vi "情景列表删除.vi"(9 "删除节点":string, 10 "父节点（场景）":string, 11 "模式列表":T1(array[cluster])) -> (3 "模式列表-output":T1(array[cluster]))   [LabVIEW 2019]
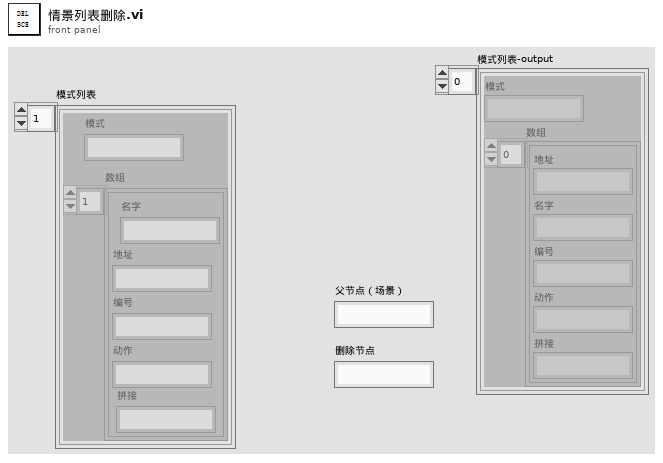
[diagram p1: front panel]
types:
  T1 = cluster{"模式":string, "数组":cluster{"地址":string, "名字":string, "编号":string, "动作":string, "拼接":string}[]}[]
  T2 = cluster{"模式":string, "数组":cluster{"地址":string, "名字":string, "编号":string, "动作":string, "拼接":string}[]}
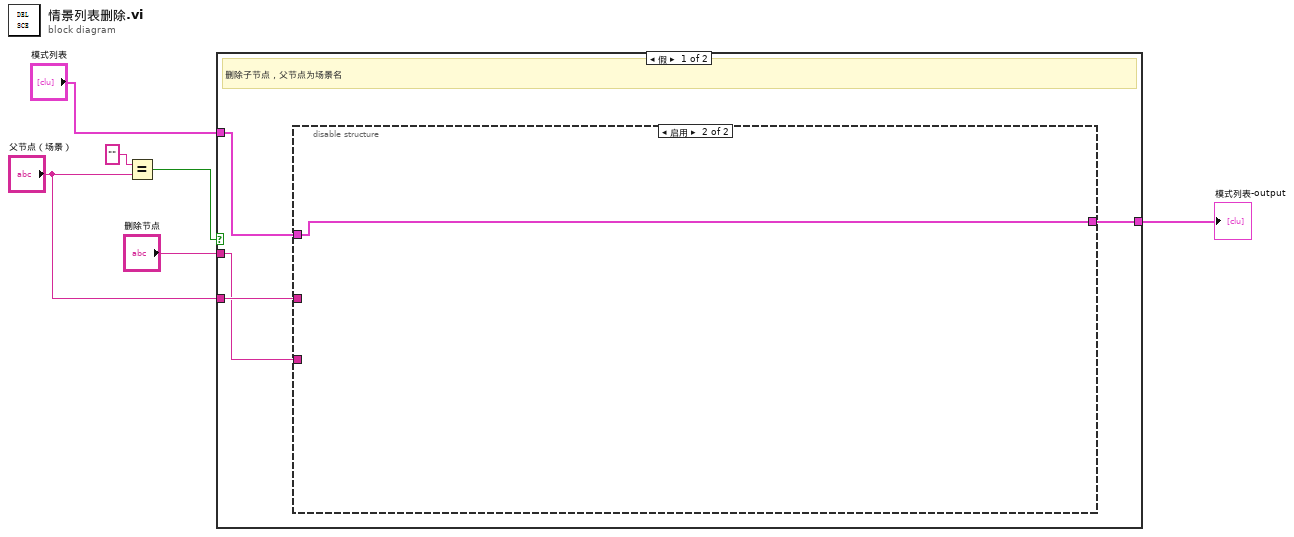
[diagram p0: block diagram]
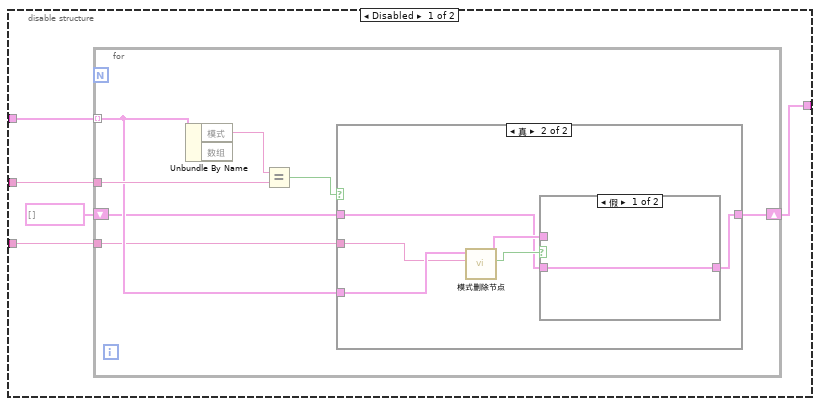
[diagram p2: hidden frame]
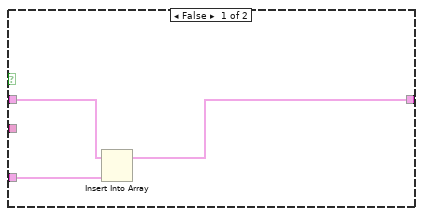
[diagram p3: hidden frame]
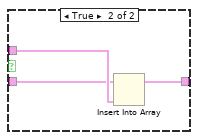
[diagram p4: hidden frame]
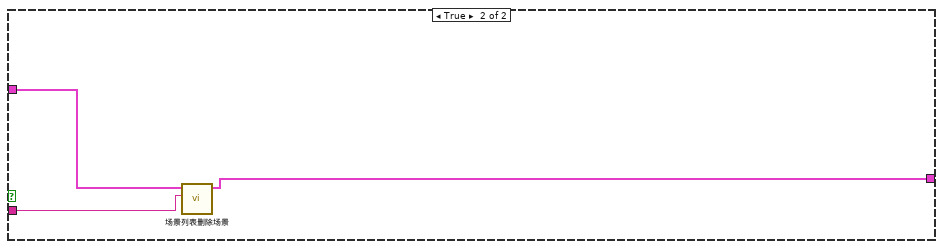
[diagram p5: hidden frame]
diagram:
  n1 = Equal?(x="", y="父节点（场景）") -> (x = y?=w5:bool)
  n2 = case shown="假" w5 {
    tunnel: "模式列表" -> [w10 w39]
    tunnel: "删除节点" -> [w8 w38]
    tunnel: [w7 w37] -> w2
    tunnel: "父节点（场景）" -> [w9 _]
    frame False {
      # "删除子节点，父节点为场景名"
      n3 = disable-structure shown="启用" {
        disable-tunnel: w10 -> [w15 w36]
        disable-tunnel: w9 -> [w14 _]
        disable-tunnel: w8 -> [w12 _]
        disable-tunnel: [w11 w36] -> w7
        frame Disabled {
          n4 = for {
            tunnel: w15 -> [w19] mode=indexing
            tunnel: w14 -> [w21]
            shift-right: [w18] -> w11
            shift-left: T1 [] -> [w17]
            tunnel: w12 -> [w16]
            n5 = Unbundle By Name(w19) -> ("模式"=w22:string)  [unwired: 1 out]
            n6 = Equal?(x=w22, y=w21) -> (x = y?=w20:bool)
            n7 = case shown="真" w20 {
              tunnel: w19 -> [w25 w31]
              tunnel: [w24 w27] -> w18
              tunnel: w17 -> [w23 w26]
              tunnel: w16 -> [_ w30]
              frame False {
                n8 = Insert Into Array(array=w23, new element=w25) -> (w24:T1)  [unwired: 1 in]
              }
              frame True {
                n9 = call "模式删除节点.vi"("名字"=w30, "模式"=w31) -> ("模式合法"=w29:bool, "模式-output"=w28:T2)  [unwired: 8 in]
                n10 = case shown="假" w29 {
                  tunnel: w28 -> [_ w35]
                  tunnel: [w32 w34] -> w27
                  tunnel: w26 -> [w32 w33]
                  frame False {
                  }
                  frame True {
                    n11 = Insert Into Array(array=w33, new element=w35) -> (w34:T1)  [unwired: 1 in]
                  }
                }
              }
            }
          }
        }
        frame Enabled {
        }
      }
    }
    frame True {
      n12 = call "场景列表删除场景.vi"("场景"=w38, "模式列表"=w39) -> ("模式列表-output"=w37:T1)  [unwired: 9 in]
    }
  }
  "模式列表-output" <- w2
